vi "Init FreeType.vi"(8 "error in (no error)":errorcluster) -> (0 "error out":errorcluster, 3 "library":i64)   [LabVIEW 2023, in "Freetype Drawer.lvlib"]
uses:
  Freetype Drawer.lvlib
  libfreetype.dll
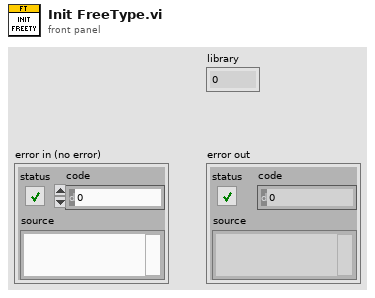
[diagram p1: front panel]
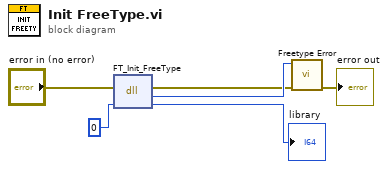
[diagram p0: block diagram]
diagram:
  n1 = dll-call lib="E:/Labview/LV 2023/Libs/LV Symbol/Freetype Drawer/Wrappers/libfreetype.dll" fn="FT_Init_FreeType"(error in="error in (no error)", "library"=i64 0) -> (error out=w3:errorcluster, "error"=w6:i32, "library"=→"library":i64)  [unwired: 2 in, 1 out]
  n2 = call "Freetype Error.vi"("error in (no error)"=w3, "Error"=w6) -> ("error out"=→"error out":errorcluster)  [unwired: 9 in]
